vi "Joystick Override.vi"(10 "Aircraft Update Rate (Hz)":dbl=30.0, 11 "Instance Details":T1) -> ()   [LabVIEW 2014]
uses:
  Ground Station to Aircraft Coms/SubVI/Aircraft Data Router/Controls/Known Aircraft.ctl
  Ground Station to Aircraft Coms/SubVI/Hardware Driver/Controls/Coms Driver Interface.ctl
  Telemetry/Controls/Telemetry Connection Type.ctl
  <vilib>/httpClient/ClientHandle.ctl
  Application Support/Stop Button/SubVI/Get Stop Button Status.vi
  Joystick/FGVs/Joystick Input/Method VIs/Get Joystick Input.vi
  Commands/MAV_CMD Sub VI/MAV_CMD_COMPONENT_ARM_DISARM.vi
  Joystick/FGVs/Joystick Flight Mode/Method VIs/Get Joystick Flight Mode.vi
  <vilib>/httpClient/LabVIEWHTTPClient.lvlib
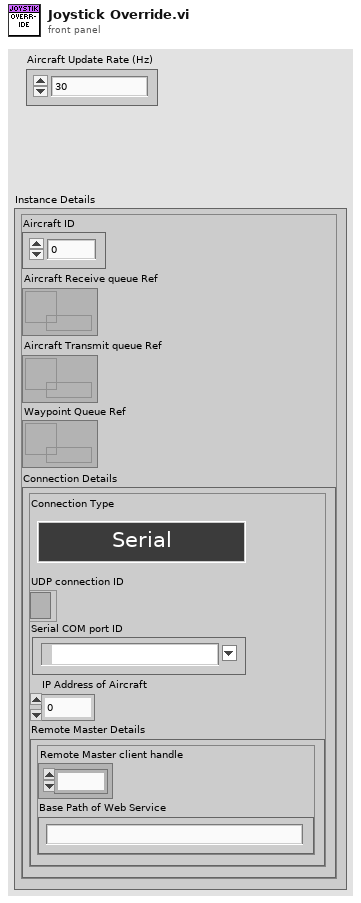
[diagram p1: front panel]
types:
  T1 = typedef "Known Aircraft.ctl" = cluster{"Aircraft ID":u8, "Aircraft Receive queue Ref":refnum<queue>, "Aircraft Transmit queue Ref":refnum<queue>, "Waypoint Queue Ref":refnum<queue>, "Connection Details":T2}
  T2 = typedef "Coms Driver Interface.ctl" = cluster{"Connection Type":T3, "UDP connection ID":refnum<k16>, "Serial COM port ID":refnum<visa-resource-name>, "IP Address of Aircraft":u32, "Remote Master Details":cluster{"Remote Master client handle":T4, "Base Path of Web Service":string}}
  T3 = typedef "Telemetry Connection Type.ctl" = enum16{"Serial", "UDP", "Remote Master"}
  T4 = typedef "LabVIEWHTTPClient.lvlib/ClientHandle.ctl" = refnum<k1>
  T5 = typedef "Joystick Input.ctl" = cluster{"Roll (%)":dbl, "Pitch (%)":dbl, "Yaw (%)":dbl, "Throttle (%)":dbl, "Brake":bool, "Emergency Stop":bool, "Arm":bool, "Disarm":bool}
  T6 = cluster{"chan1_raw":u16, "chan2_raw":u16, "chan3_raw":u16, "chan4_raw":u16, "chan5_raw":u16, "chan6_raw":u16, "chan7_raw":u16, "chan8_raw":u16, "target_system":u8, "target_component":u8}
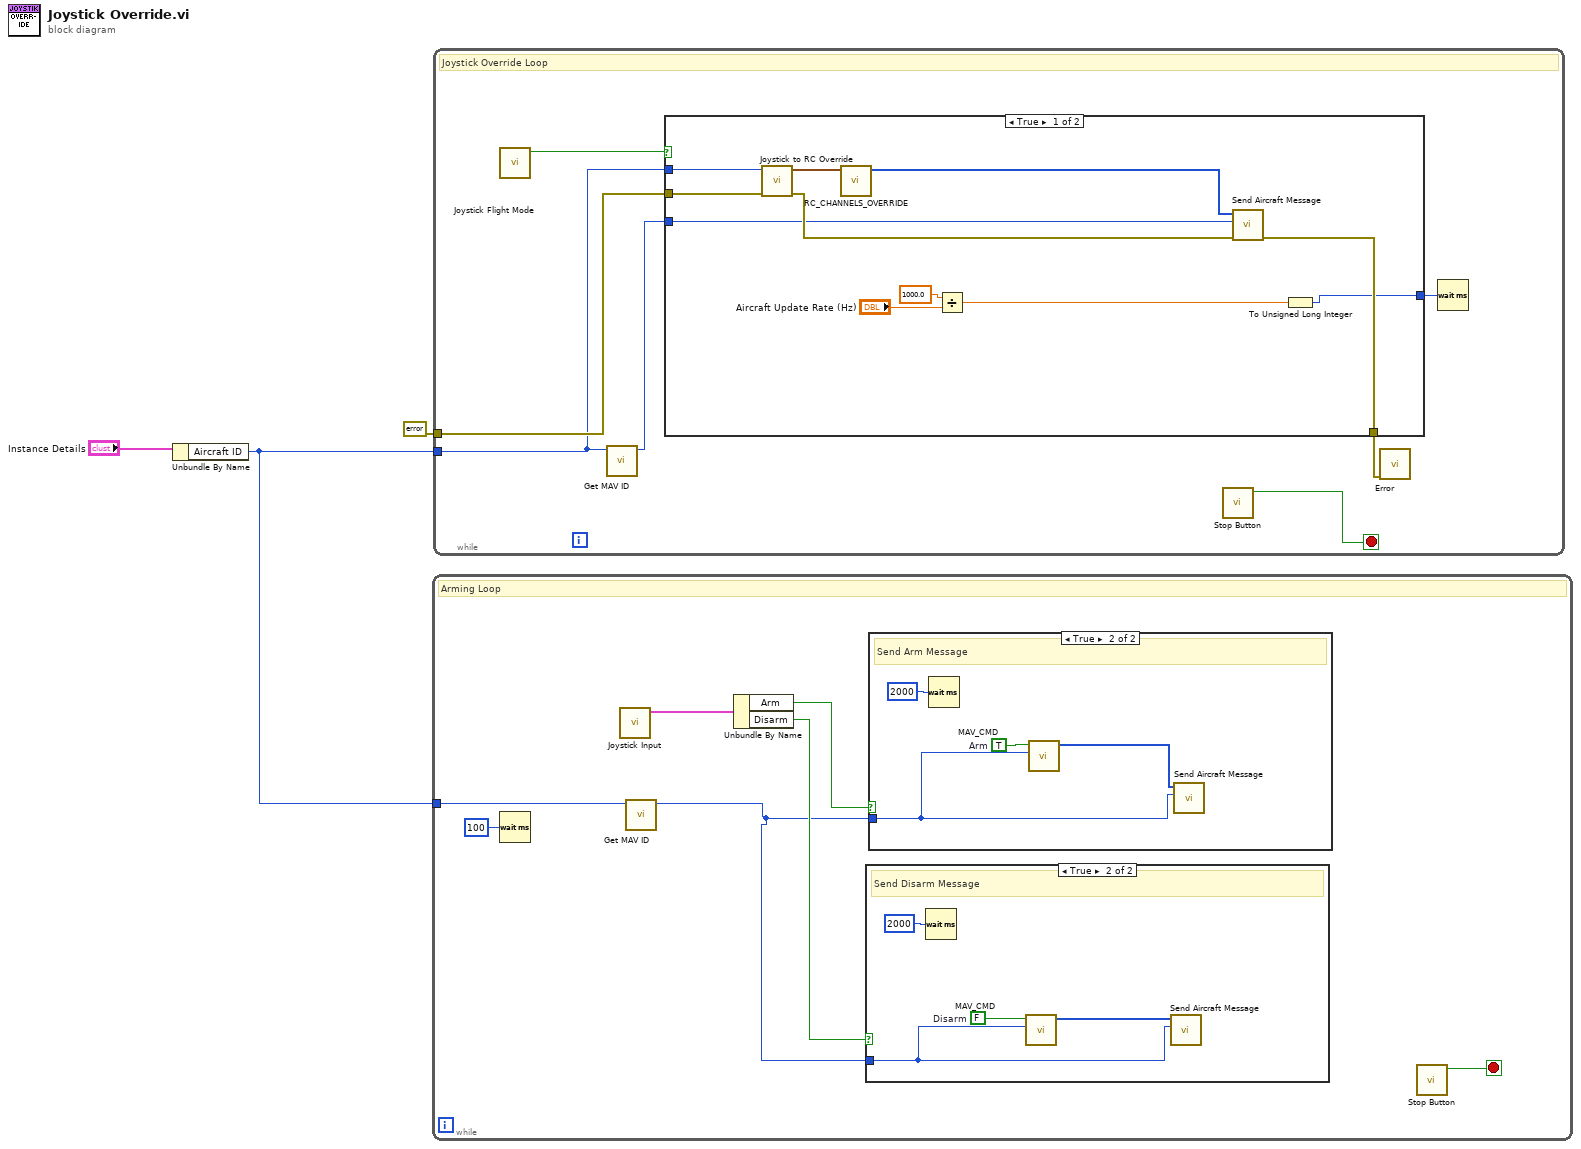
[diagram p0: block diagram]
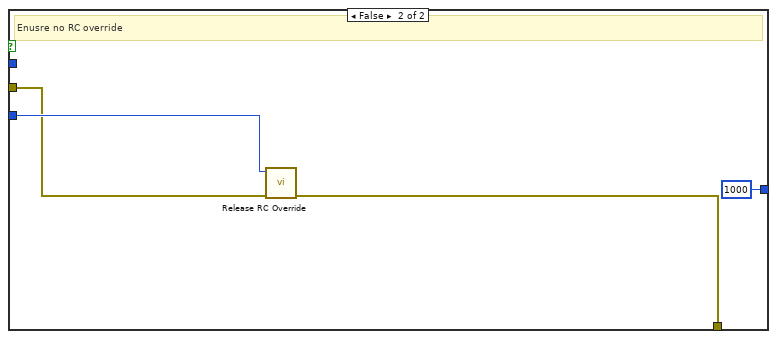
[diagram p4: hidden frame]
diagram:
  n1 = Unbundle By Name("Instance Details") -> ("Aircraft ID"=w1:u8)
  n2 = while {
    tunnel: w1 -> [w8]
    stop <- w9 stop-if-true
    # "Arming Loop"
    n3 = Wait (ms)(milliseconds to wait=u32 100) -> ()  [unwired: 1 out]
    n4 = call-poly "Joystick Input.vi"() -> ("Joystick Input Out"=w7:T5)  [unwired: 11 in]
    n5 = call "Get MAV ID.vi"("Aircraft Index"=w8) -> ("Aircraft ID"=w4:u8)  [unwired: 9 in, 1 out]
    n6 = Unbundle By Name(w7) -> ("Arm"=w5:bool, "Disarm"=w6:bool)
    n7 = case shown="True" w6 {
      tunnel: w4 -> [_ w15]
      frame False {
      }
      frame True {
        w18 = FALSE  # Disarm
        # "Send Disarm Message"
        n8 = Wait (ms)(milliseconds to wait=u32 2000) -> ()  [unwired: 1 out]
        n9 = call-poly "MAV_CMD.vi"("Target System and Target Component"=w15, "ARM(T)/DISARM(F)"=w18) -> ("MAVLink Message"=w17:u8[])  [unwired: 9 in]
        n10 = call "Send Aircraft Message.vi"("Aircraft ID"=w15, "MAVLink Message"=w17) -> ()  [unwired: 9 in, 1 out]
      }
    }
    n11 = case shown="True" w5 {
      tunnel: w4 -> [_ w11]
      frame False {
      }
      frame True {
        w14 = TRUE  # Arm
        # "Send Arm Message"
        n12 = Wait (ms)(milliseconds to wait=u32 2000) -> ()  [unwired: 1 out]
        n13 = call-poly "MAV_CMD.vi"("Target System and Target Component"=w11, "ARM(T)/DISARM(F)"=w14) -> ("MAVLink Message"=w13:u8[])  [unwired: 9 in]
        n14 = call "Send Aircraft Message.vi"("Aircraft ID"=w11, "MAVLink Message"=w13) -> ()  [unwired: 9 in, 1 out]
      }
    }
    n15 = call-poly "Stop Button.vi"() -> ("Stop ButtonOut"=w9:bool)  [unwired: 10 in, 1 out]
  }
  n16 = while {
    tunnel: w1 -> [w22]
    tunnel: errorcluster {"status"=FALSE, "code"=0, "source"=""} ("error in (no error)") -> [w23]
    stop <- w25 stop-if-true
    # "Joystick Override Loop"
    n17 = call-poly "Joystick Flight Mode.vi"() -> ("Enabled?"=w20:bool)  [unwired: 11 in]
    n18 = call "Get MAV ID.vi"("Aircraft Index"=w22) -> ("Aircraft ID"=w21:u8)  [unwired: 9 in, 1 out]
    n19 = case shown="True" w20 {
      tunnel: [w35 w37] -> w24
      tunnel: w23 -> [w33 w38]
      tunnel: w22 -> [w31 _]
      tunnel: w21 -> [w30 w39]
      tunnel: [w26 u32 1000] -> w19
      frame True {
        n20 = call "Joystick to RC Override.vi"("Error In"=w33, "Aircraft ID"=w31) -> ("Error Out"=w32:errorcluster, "output cluster"=w34:T6)  [unwired: 8 in]
        n21 = call "RC_CHANNELS_OVERRIDE.vi"("Payload"=w34) -> ("MAVLink Message"=w36:u8[])  [unwired: 10 in]
        n22 = Divide(x=1000.0, y="Aircraft Update Rate (Hz)") -> (x/y=w29:dbl)
        n23 = call "Send Aircraft Message.vi"("error in (no error)"=w32, "Aircraft ID"=w30, "MAVLink Message"=w36) -> ("error out"=w35:errorcluster)  [unwired: 8 in]
        n24 = To Unsigned Long Integer(number=w29) -> (unsigned 32bit integer=w26:u32)
      }
      frame False {
        # "Enusre no RC override"
        n25 = call "Release RC Override.vi"("error in (no error)"=w38, "Aircraft ID"=w39) -> ("error out"=w37:errorcluster)  [unwired: 9 in]
      }
    }
    n26 = call-poly "Stop Button.vi"() -> ("Stop ButtonOut"=w25:bool)  [unwired: 10 in, 1 out]
    n27 = call "Error.vi"("Error In"=w24) -> ()  [unwired: 10 in, 1 out]
    n28 = Wait (ms)(milliseconds to wait=w19) -> ()  [unwired: 1 out]
  }
